vi "First Step.vi"(8 "error in (no error)":errorcluster, 11 "Magna Voltage Scan.lvclass in":refnum<class "Magna Voltage Scan.lvclass">) -> (0 "error out":errorcluster, 2 "Current Position":dbl, 3 "Magna Voltage Scan.lvclass out":refnum<class "Magna Voltage Scan.lvclass">)   [LabVIEW 2017, in "Magna Voltage Scan.lvclass"]
doc: "(Dynamic) Reset the instrument and prepare to scan. Go to step #0 - the first step. If desired, the scanner may do this in a different way than usual (i.e. by preparing to move a long distance, or reset to home position.)"
uses:
  Magna Voltage Scan.lvclass
  Instruments/Magna-Power Power Supply/Magna Power.lvclass
  C:/LabVIEW-programs-dev/Instruments/Utility Classes/Scannable/Scannable.lvclass
  Magna Voltage Scan.lvclass/Magna Voltage Scan.ctl
  Instruments/Magna-Power Power Supply/Magna Power Constants.vi
  Scanner/Scanner.lvclass
  <vilib>/gmath/NI_Gmath.lvlib
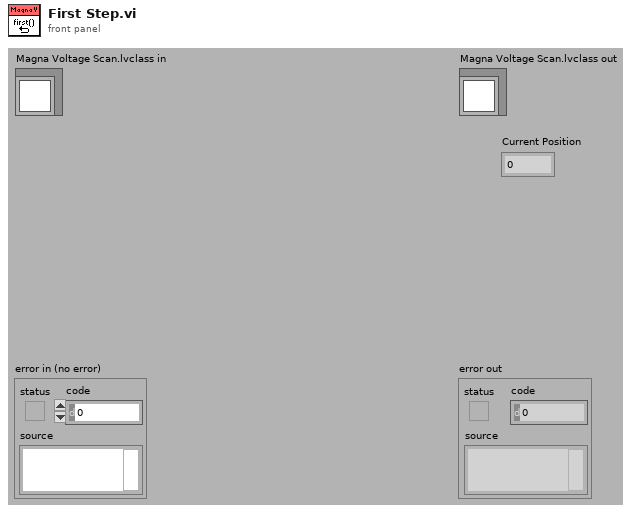
[diagram p1: front panel]
types:
  T1 = cluster{"Magna Voltage":dbl[], "Magna Current":dbl[], "Magnetic Field":dbl[], "Fluke Voltage":dbl[]}
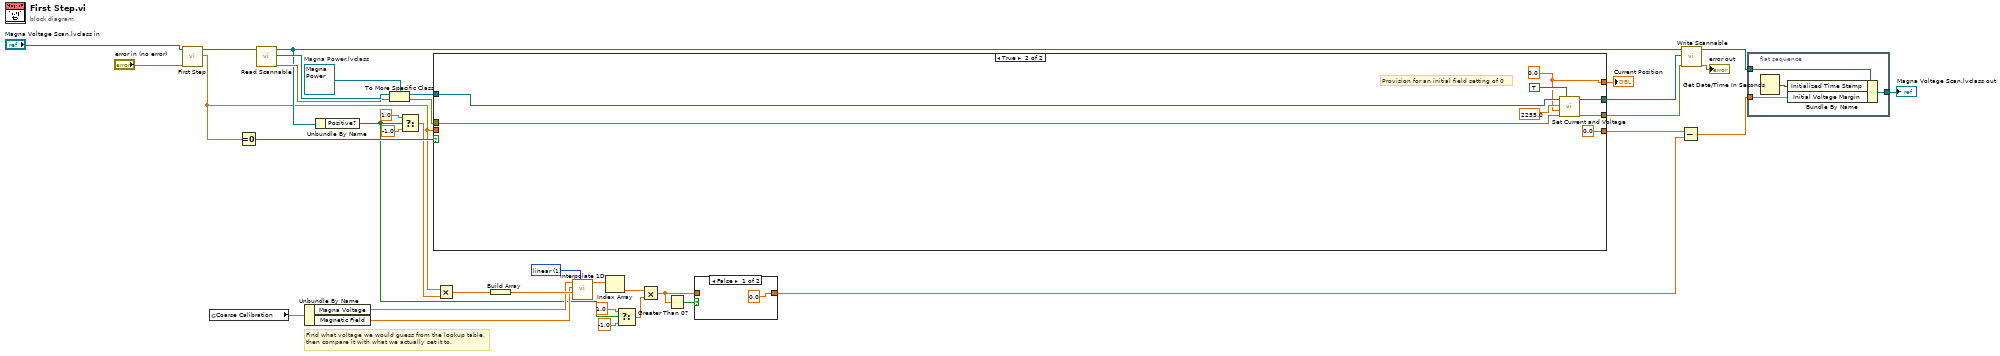
[diagram p0: block diagram]
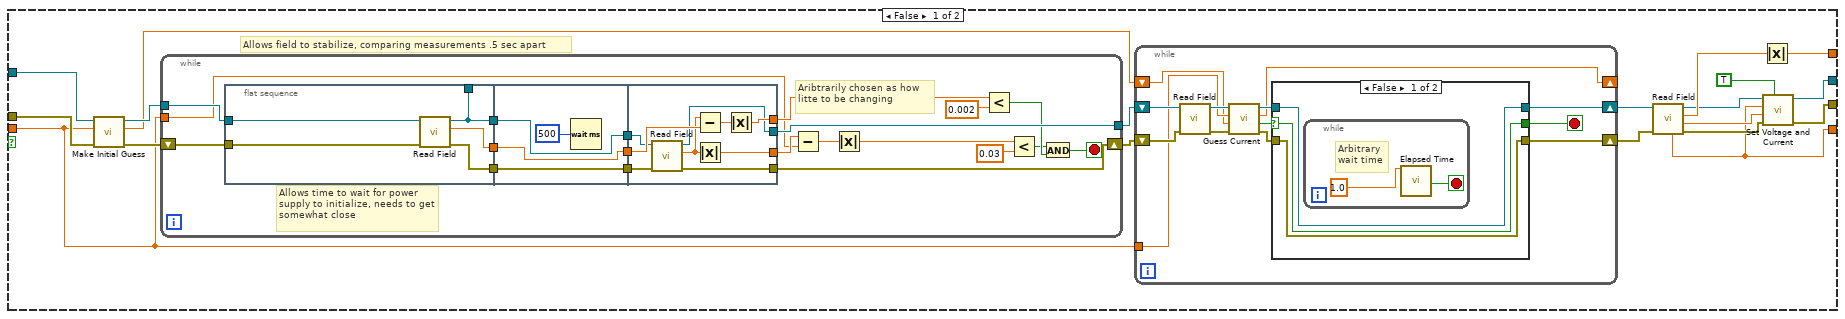
[diagram p3: hidden frame]
diagram:
  w25 = 1 items=["nearest", "linear", "spline", "cubic Hermite", "Lagrange"] ("method")
  w35 = refnum<class "Magna Power.lvclass"> refnum  # Magna Power.lvclass
  # "Find what voltage we would guess from the lookup table, then compare it with what we actually set it to."
  n1 = call-parent "First Step.vi"("error in (no error)"="error in (no error)", "Scanner.lvclass in"="Magna Voltage Scan.lvclass in") -> ("Current Position"=w4:dbl, "Scanner.lvclass out"=w5:refnum<class "Magna Voltage Scan.lvclass">)  [unwired: 7 in, 1 out]
  n2 = global read "Magna Power Constants.vi" "Coarse Calibration"() -> (w26:T1)
  n3 = Equal To 0?(x=w4) -> (x = 0?=w27:bool)
  n4 = call-dynamic "Read Scannable.vi"("Scanner.lvclass in"=w5) -> ("error out"=w33:errorcluster, "Scannable.lvclass"=w34:refnum<class "Scannable.lvclass">, "Scanner.lvclass out"=w11:refnum<class "Magna Voltage Scan.lvclass">)  [unwired: 8 in]
  n5 = Unbundle By Name(w26) -> ("Magna Voltage"=w21:dbl[], "Magnetic Field"=w22:dbl[])
  n6 = Unbundle By Name(w11) -> ("Positive?"=w10:bool)
  n7 = To More Specific Class(target class=w35, reference=w34, error in=w33) -> (specific class reference=w31:refnum<class "Magna Power.lvclass">, error out=w32:errorcluster)
  n8 = Select(t=1.0, s=w10, f=-1.0) -> (s? t:f=w12:dbl)
  n9 = case shown="True" w27 {
    tunnel: w32 -> [w52 w123]
    tunnel: w31 -> [w51 w122]
    tunnel: w4 -> [w50 _]
    tunnel: [w48 w116] -> w3
    tunnel: [w40 w120] -> w30
    tunnel: [w41 w119] -> w29
    tunnel: [w39 0.0 ("Numeric")] -> w8
    frame False {
      # "Allows field to stabilize, comparing measurements .5 sec apart"
      n10 = call "Make Initial Guess.vi"("error in (no error)"=w52, "Desired Field"=w50, "Magna Power in"=w51) -> ("error out"=w53:errorcluster, "First guess"=w49:dbl, "Magna Power out"=w54:refnum<class "Magna Power.lvclass">)  [unwired: 6 in]
      n11 = while {
        shift-right: [w91] -> w56
        shift-left: w53 -> [w97]
        tunnel: w54 -> [w89]
        tunnel: [w86] -> w55
        tunnel: w50 -> [w82]
        stop <- w85 stop-if-true
        # "Aribtrarily chosen as how litte to be changing"
        # "Allows time to wait for power supply to initialize, needs to get somewhat close"
        n12 = flat-sequence {
          tunnel: w97 -> [w102]
          tunnel: [w101] -> w95
          tunnel: [w100] -> w93
          tunnel: w89 -> [w99]
          tunnel: [w98] -> w87
          tunnel: [w98] -> _
          tunnel: [w105] -> w96
          tunnel: w95 -> [w105]
          tunnel: [w104] -> w94
          tunnel: w93 -> [w104]
          tunnel: [w103] -> w88
          tunnel: w87 -> [w103]
          tunnel: w96 -> [w115]
          tunnel: w94 -> [w113]
          tunnel: [w112] -> w90
          tunnel: [w111] -> w91
          tunnel: w88 -> [w109]
          tunnel: [w110] -> w86
          tunnel: [w107] -> w83
          frame #0 {
            n13 = call "Read Field.vi"("error in (no error)"=w102, "Magna Power in"=w99) -> ("error out"=w101:errorcluster, "Field (T)"=w100:dbl, "Magna Power out"=w98:refnum<class "Magna Power.lvclass">)  [unwired: 5 in, 2 out]
          }
          frame #1 {
            n14 = Wait (ms)(milliseconds to wait=u32 500) -> ()  [unwired: 1 out]
          }
          frame #2 {
            n15 = call "Read Field.vi"("error in (no error)"=w115, "Magna Power in"=w109) -> ("error out"=w111:errorcluster, "Field (T)"=w108:dbl, "Magna Power out"=w110:refnum<class "Magna Power.lvclass">)  [unwired: 5 in, 2 out]
            n16 = Subtract(x=w108, y=w113) -> (x-y=w114:dbl)
            n17 = Absolute Value(x=w108) -> (abs(x)=w107:dbl)
            n18 = Absolute Value(x=w114) -> (abs(x)=w112:dbl)
          }
        }
        n19 = Subtract(x=w83, y=w82) -> (x-y=w81:dbl)
        n20 = Absolute Value(x=w81) -> (abs(x)=w80:dbl)
        n21 = Less?(x=w90, y=0.002) -> (x < y?=w84:bool)
        n22 = Less?(x=w80, y=0.03) -> (x < y?=w78:bool)
        n23 = And(x=w78, y=w84) -> (x .and. y?=w85:bool)
      }
      n24 = while {
        shift-right: [w65] -> w46
        shift-left: w56 -> [w69]
        shift-right: [w60] -> w47
        shift-left: w55 -> [w64]
        tunnel: w50 -> [w59]
        shift-right: [w57] -> _
        shift-left: w49 -> [w58]
        stop <- w62 stop-if-true
        n25 = call "Read Field.vi"("error in (no error)"=w69, "Magna Power in"=w64) -> ("error out"=w68:errorcluster, "Magna Power out"=w61:refnum<class "Magna Power.lvclass">)  [unwired: 5 in, 3 out]
        n26 = call "Guess Current.vi"("error in (no error)"=w68, "Current guess"=w58, "Desired Field"=w59, "Magna Power in"=w61) -> ("error out"=w66:errorcluster, "Stop?"=w67:bool, "New guess"=w57:dbl, "Magna Power out"=w63:refnum<class "Magna Power.lvclass">)  [unwired: 4 in]
        n27 = case shown="False" w67 {
          selector: w67 -> [w72 w77]
          tunnel: [w72 w77] -> w62
          tunnel: w66 -> [w70 w75]
          tunnel: [w70 w75] -> w65
          tunnel: w63 -> [w71 w76]
          tunnel: [w71 w76] -> w60
          frame False {
            n28 = while {
              stop <- w73 stop-if-true
              # "Arbitrary\nwait time"
              n29 = call "Elapsed Time"("Time Target (s)"=1.0) -> ("Time has Elapsed"=w73:bool)  [unwired: 11 in, 7 out]
            }
          }
          frame True {
          }
        }
      }
      n30 = call "Read Field.vi"("error in (no error)"=w46, "Magna Power in"=w47) -> ("error out"=w45:errorcluster, "Current"=w44:dbl, "Field (T)"=w43:dbl, "Magna Power out"=w42:refnum<class "Magna Power.lvclass">, "Voltage"=w39:dbl)  [unwired: 5 in]
      n31 = Absolute Value(x=w43) -> (abs(x)=w48:dbl)
      n32 = call "Set Voltage and Current.vi"("Wait?"=TRUE, "error in (no error)"=w45, "Current Limit"=w44, "Voltage Limit"=w39, "Magna Power in"=w42) -> ("error out"=w40:errorcluster, "Magna Power out"=w41:refnum<class "Magna Power.lvclass">)  [unwired: 5 in]
    }
    frame True {
      w116 = 0.0 ("Current Limit")
      # "Provision for an initial field setting of 0"
      n33 = call "Set Current and Voltage.vi"("Wait?"=TRUE, "error in (no error)"=w123, "Current Limit"=w116, "Voltage Limit"=2255.0, "Magna Power in"=w122) -> ("error out"=w120:errorcluster, "Magna Power out"=w119:refnum<class "Magna Power.lvclass">)  [unwired: 5 in]
    }
  }
  "Current Position" <- w3
  n34 = Multiply(x=w4, y=w12) -> (x*y=w9:dbl)
  n35 = Build Array(w9) -> (w24:dbl[])
  n36 = call <vilib>:"Interpolate 1D.vi"("method"=w25, "xi"=w24, "X"=w22, "Y"=w21) -> ("yi"=w23:dbl[])  [unwired: 5 in, 2 out]
  n37 = Index Array(array=w23) -> (element=w17:dbl)  [unwired: 1 in]
  n38 = Select(t=1.0, s=w10, f=-1.0) -> (s? t:f=w16:dbl)
  n39 = Multiply(x=w17, y=w16) -> (x*y=w15:dbl)
  n40 = Greater Than 0?(x=w15) -> (x > 0?=w20:bool)
  n41 = case shown="False" w20 {
    tunnel: [0.0 ("Numeric") w125] -> w7
    tunnel: w15 -> [_ w125]
    frame False {
    }
    frame True {
    }
  }
  n42 = Subtract(x=w8, y=w7) -> (x-y=w6:dbl)
  n43 = call-dynamic "Write Scannable.vi"("error in (no error)"=w30, "Scannable.lvclass"=w29, "Scanner.lvclass in"=w11) -> ("error out"=→"error out":errorcluster, "Scanner.lvclass out"=w28:refnum<class "Magna Voltage Scan.lvclass">)  [unwired: 7 in]
  n44 = flat-sequence {
    tunnel: w28 -> [w128]
    tunnel: [w127] -> w2
    tunnel: w6 -> [w126]
    frame #0 {
      n45 = Get Date/Time In Seconds() -> (seconds since 1Jan1904=w129:timestamp)
      n46 = Bundle By Name(cluster=w128, "Initialized Time Stamp"=w129, "Initial Voltage Margin"=w126) -> (w127:refnum<class "Magna Voltage Scan.lvclass">)
    }
  }
  "Magna Voltage Scan.lvclass out" <- w2
